vi "Configure Hardware.vi"(8 "error in (no error)":errorcluster, 10 "Active_Profile":T1, 11 "Hardware Resources in":T2) -> (0 "error out":errorcluster, 3 "Hardware Resources out":T2)   [LabVIEW 2026, in "Acquisition.lvlib"]
doc: "Configure the hardware."
uses:
  Acquisition.lvlib
  <vilib>/DAQmx/configure/timing.llb/DAQmx Timing (Sample Clock).vi
  Hardware Configuration.ctl
  controls/Vibration_Profile.ctl
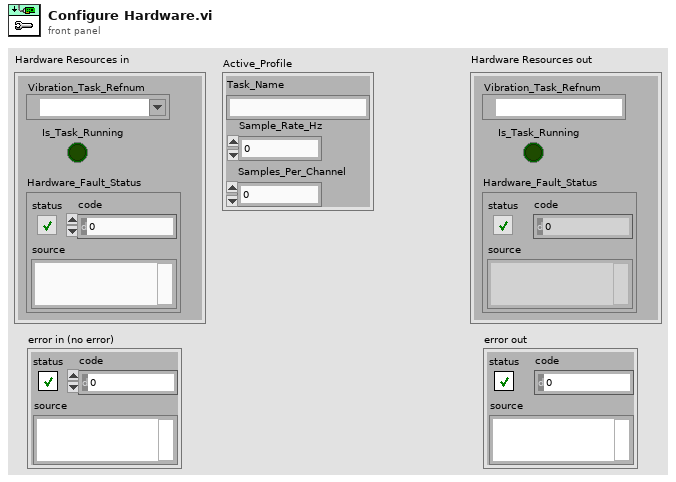
[diagram p1: front panel]
types:
  T1 = typedef "Vibration_Profile.ctl" = cluster{"Task_Name":string, "Sample_Rate_Hz":dbl, "Samples_Per_Channel":i32}
  T2 = typedef "Acquisition.lvlib/Hardware Configuration.ctl" = cluster{"Vibration_Task_Refnum":refnum<k21>, "Is_Task_Running":bool, "Hardware_Fault_Status":errorcluster}
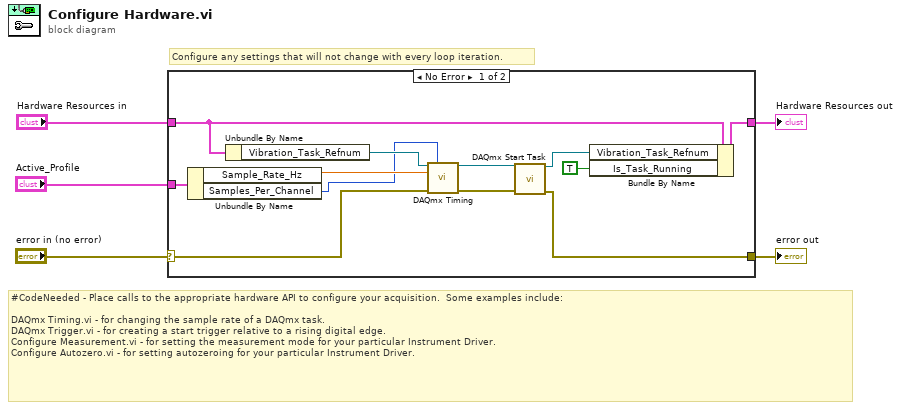
[diagram p0: block diagram]
diagram:
  # "Configure any settings that will not change with every loop iteration."
  # "#CodeNeeded - Place calls to the appropriate hardware API to configure your acquisition.  Some examples include:\n\nDAQmx Timing.vi - for changing the sample rate of a DAQmx task.\nDAQmx Trigger.vi - for creating a start trigger relative to a rising digital edge.\nConfigure Measurement.vi - for setting the measurement mode for your particular Instrument Driver.\nConfigure Autozero.vi - for setting autozeroing for your particular Instrument Driver."
  n1 = case shown="No Error" "error in (no error)" {
    selector: "error in (no error)" -> [w14 w18]
    tunnel: [w9 w18] -> w4
    tunnel: "Hardware Resources in" -> [w16 w19]
    tunnel: [w17 w19] -> w2
    tunnel: "Active_Profile" -> [w13 _]
    frame No Error {
      n2 = Unbundle By Name(w13) -> ("Sample_Rate_Hz"=w12:dbl, "Samples_Per_Channel"=w11:i32)
      n3 = Unbundle By Name(w16) -> ("Vibration_Task_Refnum"=w15:refnum<k21>)
      n4 = call-poly <vilib>:"DAQmx Timing.vi"("task/channels in"=w15, "sample mode"=w11, "rate"=w12, "error in"=w14) -> ("task out"=w8:refnum<k21>, "error out"=w10:errorcluster)  [unwired: 10 in]
      n5 = call <vilib>:"DAQmx Start Task.vi"("task/channels in"=w8, "error in"=w10) -> ("task out"=w7:refnum<k21>, "error out"=w9:errorcluster)  [unwired: 12 in]
      n6 = Bundle By Name(cluster=w16, "Vibration_Task_Refnum"=w7, "Is_Task_Running"=TRUE) -> (w17:T2)
    }
    frame Error {
    }
  }
  "Hardware Resources out" <- w2
  "error out" <- w4
